vi "Read Single Current Measurement.vi"(8 "error in (no error)":errorcluster, 10 "Single Current Measurement Type (0:DC)":u16(ring) items=["DC", "AC", "AC+DC", "Crest Factor", "Current Harmonic THD", "Neutral DC", "Neutral AC", "Neutral ACDC"], 11 "VISA resource name":refnum<visa-resource-name>) -> (0 "error out":errorcluster, 2 "Current Measurement":dbl format="%#_10g", 3 "VISA resource name out":refnum<visa-resource-name>)   [LabVIEW 2013, in "California Instruments iX Series.lvlib"]
doc: "Reads single current measurement by user selected measurement type."
uses:
  <instrlib>/California Instruments iX Series/California Instruments iX Series.lvlib
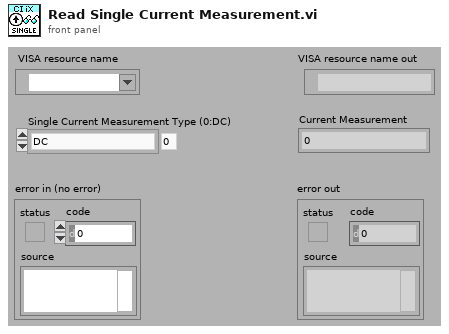
[diagram p1: front panel]
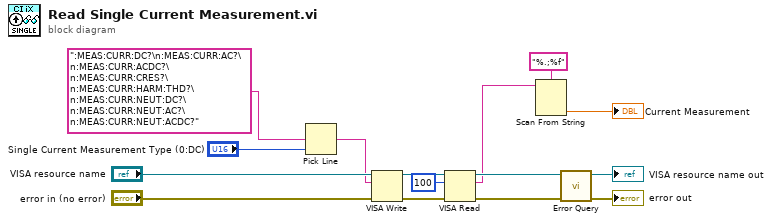
[diagram p0: block diagram]
diagram:
  n1 = Pick Line(multi-line string=":MEAS:CURR:DC?\n:MEAS:CURR:AC?\n:MEAS:CURR:ACDC?\n:MEAS:CURR:CRES?\n:MEAS:CURR:HARM:THD?\n:MEAS:CURR:NEUT:DC?\n:MEAS:CURR:NEUT:AC?\n:MEAS:CURR:NEUT:ACDC?", line index="Single Current Measurement Type (0:DC)") -> (output string=w1:string)  [unwired: 1 in]
  n2 = VISA Write(VISA resource name="VISA resource name", write buffer=w1, error in (no error)="error in (no error)") -> (VISA resource name out=w11:refnum<visa-resource-name>, error out=w10:errorcluster)  [unwired: 1 out]
  n3 = VISA Read(VISA resource name=w11, byte count=u32 100, error in (no error)=w10) -> (VISA resource name out=w9:refnum<visa-resource-name>, read buffer=w5:string, error out=w8:errorcluster)  [unwired: 1 out]
  n4 = Scan From String(format string="%.;%f", input string=w5) -> (output 1=→"Current Measurement":dbl)  [unwired: 3 in, 3 out]
  n5 = call <instrlib>:"Error Query.vi"("error in (no error)"=w8, "VISA resource name"=w9) -> ("error out"=→"error out":errorcluster, "VISA resource name out"=→"VISA resource name out":refnum<visa-resource-name>)  [unwired: 6 in, 2 out]
